vi "Wilcoxon Signed Rank Test.vi"   [LabVIEW 2024, in "NI_Gmath.lvlib"]
doc: "<p>Tests hypotheses about the <strong>mean</strong> of populations whose distributions are continuous and symmetric but not necessarily normal. You must <a href=\"nihelplauncher://docs/csh?context=lvcore_lvhowto_selectingdefaultinstpolyvi\">manually select the polymorphic instance</a> to use.</p>"
uses:
  NI_Gmath.lvlib
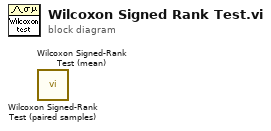
[diagram p0: block diagram]
diagram:
  n1 = call "Wilcoxon Signed-Rank Test (paired samples).vi"() -> ()  [unwired: 9 in, 3 out]
  n2 = call "Wilcoxon Signed-Rank Test (mean).vi"() -> ()  [unwired: 9 in, 3 out]
